vi "Limit Hit Safety.vi"(1 "Lower Limit":bool, 2 "Motor In":dbl, 3 "Upper Limit":bool) -> (0 "Motor Out":dbl)   [LabVIEW 2017]
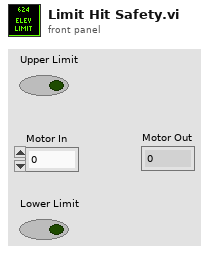
[diagram p1: front panel]
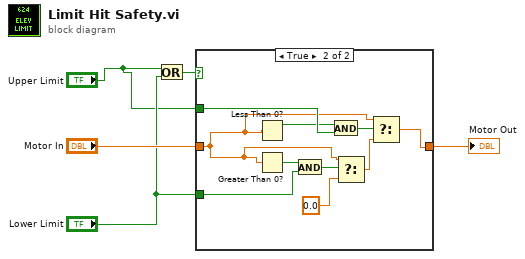
[diagram p0: block diagram]
diagram:
  n1 = Or(x="Upper Limit", y="Lower Limit") -> (x .or. y?=w5:bool)
  n2 = case shown="True" w5 {
    tunnel: "Motor In" -> [w6 w8]
    tunnel: [w6 w7] -> w3
    tunnel: "Lower Limit" -> [_ w9]
    tunnel: "Upper Limit" -> [_ w12]
    frame False {
    }
    frame True {
      n3 = Less Than 0?(x=w8) -> (x < 0?=w11:bool)
      n4 = Greater Than 0?(x=w8) -> (x > 0?=w10:bool)
      n5 = And(x=w10, y=w9) -> (x .and. y?=w14:bool)
      n6 = And(x=w11, y=w12) -> (x .and. y?=w13:bool)
      n7 = Select(t=w8, s=w14, f=0.0) -> (s? t:f=w16:dbl)
      n8 = Select(t=w8, s=w13, f=w16) -> (s? t:f=w7:dbl)
    }
  }
  "Motor Out" <- w3
